vi "Get_Printers.vi"(8 "error in (no error)":errorcluster) -> (0 "error out":errorcluster, 3 "Printers":T1(array[cluster]))   [LabVIEW 2018]
uses:
  System.Drawing
panel:
  # "1. Run the VI : all the printers should\n    appear. The default printer has his led lit.\n\n2. Set a new default printer by selecting the index\n    of the selected printer in the list.\n\nYou can also see the change of default printer in\nStart-> Printers."
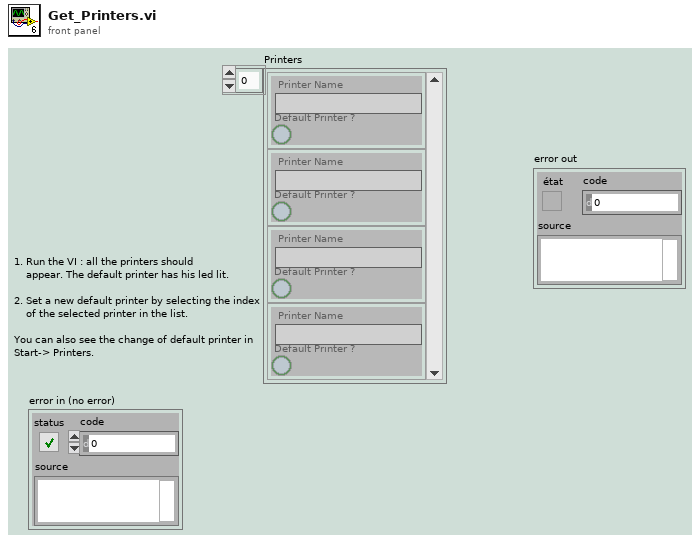
[diagram p1: front panel]
types:
  T1 = cluster{"Printer Name":string, "Default Printer ?":bool}[]
  T2 = cluster{"get_Item":string, "IsDefaultPrinter":bool}
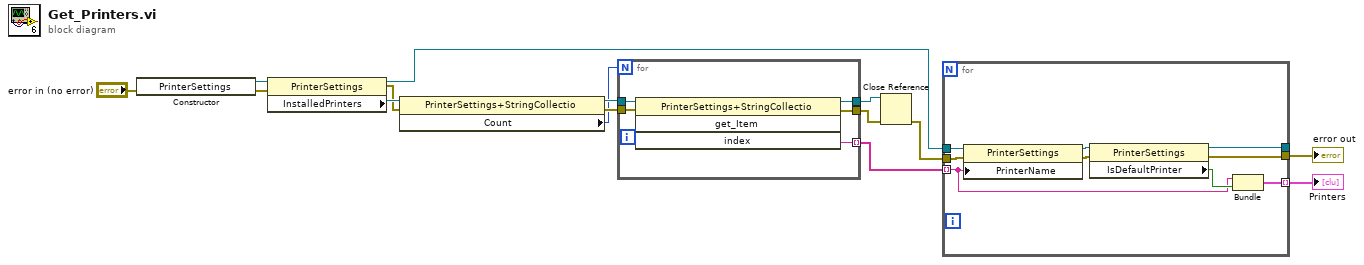
[diagram p0: block diagram]
diagram:
  n1 = constructor class="PrinterSettings"(error in="error in (no error)") -> (reference out=w9:refnum<k24>, error out=w12:errorcluster)  [unwired: 2 in, 1 out]
  n2 = property class="PrinterSettings"(reference=w9, error in=w12) -> (reference out=w6:refnum<k24>, error out=w11:errorcluster, "InstalledPrinters"=w15:refnum<k24>)
  n3 = property class="PrinterSettings+StringCollectio"(reference=w15, error in=w11) -> (reference out=w13:refnum<k24>, error out=w10:errorcluster, "Count"=w7:i32)
  n4 = for {
    N: w7 -> [_]
    tunnel: w13 -> [w21]
    tunnel: [w16] -> w5 mode=indexing
    tunnel: [w19] -> w14
    tunnel: [w18] -> w8
    tunnel: w10 -> [w17]
    i -> [w20]
    n5 = invoke class="PrinterSettings+StringCollectio" method="get_Item"(reference=w21, error in=w17, "index"=w20) -> (reference out=w19:refnum<k24>, error out=w18:errorcluster, "get_Item"=w16:string)  [unwired: 1 in, 1 out]
  }
  n6 = Close Reference(reference=w14, error in (no error)=w8) -> (error out=w2:errorcluster)
  n7 = for {
    tunnel: [w28] -> _
    tunnel: [w26] -> w4 mode=indexing
    tunnel: w6 -> [w25]
    tunnel: w5 -> [w24] mode=indexing
    tunnel: [w23] -> w3
    tunnel: w2 -> [w22]
    n8 = property class="PrinterSettings"(reference=w25, error in=w22, "PrinterName"=w24) -> (reference out=w30:refnum<k24>, error out=w29:errorcluster)
    n9 = property class="PrinterSettings"(reference=w30, error in=w29) -> (reference out=w28:refnum<k24>, error out=w23:errorcluster, "IsDefaultPrinter"=w27:bool)
    n10 = Bundle("get_Item"=w24, "IsDefaultPrinter"=w27) -> (w26:T2)  [unwired: 1 in]
  }
  "Printers" <- w4
  "error out" <- w3
